vi "From Datum.vi"(0 "Value":refnum<class "Datum.lvclass">, 1 "Key":string) -> (2 "Pair":refnum<class "Pair.lvclass">)   [LabVIEW 2018, in "Toolkit.lvlib" / "Data.lvlib" / "Pair.lvclass"]
uses:
  Pair.lvclass
  Datum/Datum.lvclass
  Pair.lvclass/Pair.ctl
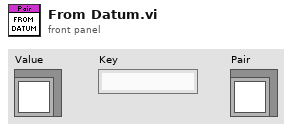
[diagram p1: front panel]
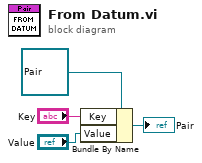
[diagram p0: block diagram]
diagram:
  n1 = Bundle By Name(cluster=refnum<class "Pair.lvclass"> refnum ("Toolkit.lvlib:Data.lvlib:Pair.lvclass"), "Key"="Key", "Value"="Value") -> (→"Pair":refnum<class "Pair.lvclass">)
